vi "Default Configuration Parameters.vi"() -> (3 "Default Configuration":T1)   [LabVIEW 2020, in "RandomNumberGenerator.lvlib" / "RandomNumberGenerator.lvclass"]
doc: "<b>Default Configuration Parameters</b>\nThis VI allows you to define default parameter values for your plugin. These defaults will be loaded by the configuration utility when you add this plugin to a configuration."
uses:
  RandomNumberGenerator.lvclass
  RandomNumberGenerator.lvclass/RandomNumberGenerator.ctl
  Configuration.ctl
panel:
  # "#via_ignore"
  # "** Updates must be made on block diagram **"
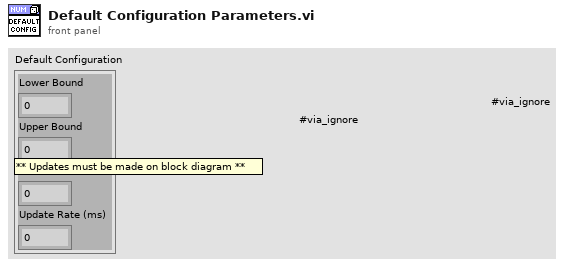
[diagram p1: front panel]
types:
  T1 = typedef "RandomNumberGenerator.lvlib/RandomNumberGenerator.lvclass/Configuration.ctl" = cluster{"Lower Bound":dbl, "Upper Bound":dbl, "# Elements":i32, "Update Rate (ms)":i32}
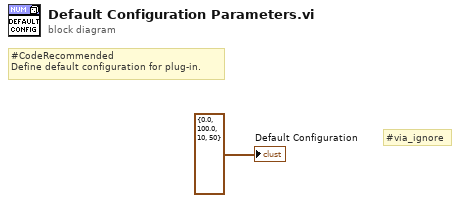
[diagram p0: block diagram]
diagram:
  # "#via_ignore"
  # "#CodeRecommended\nDefine default configuration for plug-in."
  "Default Configuration" <- T1 {"Lower Bound"=0.0, "Upper Bound"=100.0, "# Elements"=10, "Update Rate (ms)"=50} ("Default Configuration")
